vi "MGI Set Multicolumn Listbox Scrollbar.vi"(10 "Error In":errorcluster, 11 "Listbox Reference In":refnum<vi>) -> (2 "Error Out":errorcluster, 3 "Listbox Reference Out":refnum<vi>)   [LabVIEW 2016]
doc: "Show or hide the specified multicolumn listbox's horizontal and vertical scrollbar based on the listbox contents. This VI will also set the scrollbar position as necessary to ensure that some of the listbox's contents is displayed.\n\nAuthored by Shawn Walpole\nsupport@mooregoodideas.com\nwww.mooregoodideas.com\n\nCopyright (c) 2010, Moore Good Ideas, Inc.\n\nAll rights reserved.\n\nRedistribution and use in source and binary forms, with or without modification, are permitted provided that the following conditions are met:\n\n * Redistributions of source code must retain the above copyright notice, this list of conditions and the following disclaimer.\n * Redistributions in binary form must reproduce the above copyright notice, this list of conditions and the following disclaimer in the documentation and/or other materials provided with the distribution.\n * Neither the name of Moore Good Ideas, Inc. nor the names of its contributors may be used to endorse or promote products derived from this software without specific prior written permission.\n\nTHIS SOFTWARE IS PROVIDED BY THE COPYRIGHT HOLDERS AND CONTRIBUTORS \"AS IS\" AND ANY EXPRESS OR IMPLIED WARRANTIES, INCLUDING, BUT NOT LIMITED TO, THE IMPLIED WARRANTIES OF MERCHANTABILITY AND FITNESS FOR A PARTICULAR PURPOSE ARE DISCLAIMED. IN NO EVENT SHALL THE COPYRIGHT OWNER OR CONTRIBUTORS BE LIABLE FOR ANY DIRECT, INDIRECT, INCIDENTAL, SPECIAL, EXEMPLARY, OR CONSEQUENTIAL DAMAGES (INCLUDING, BUT NOT LIMITED TO, PROCUREMENT OF SUBSTITUTE GOODS OR SERVICES; LOSS OF USE, DATA, OR PROFITS; OR BUSINESS INTERRUPTION) HOWEVER CAUSED AND ON ANY THEORY OF LIABILITY, WHETHER IN CONTRACT, STRICT LIABILITY, OR TORT (INCLUDING NEGLIGENCE OR OTHERWISE) ARISING IN ANY WAY OUT OF THE USE OF THIS SOFTWARE, EVEN IF ADVISED OF THE POSSIBILITY OF SUCH DAMAGE."
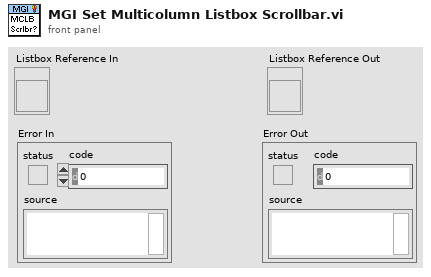
[diagram p1: front panel]
types:
  T1 = typedef "LVRowAndColumnUnsignedTypeDef.ctl" = cluster{"Row":u32, "Column":u32}
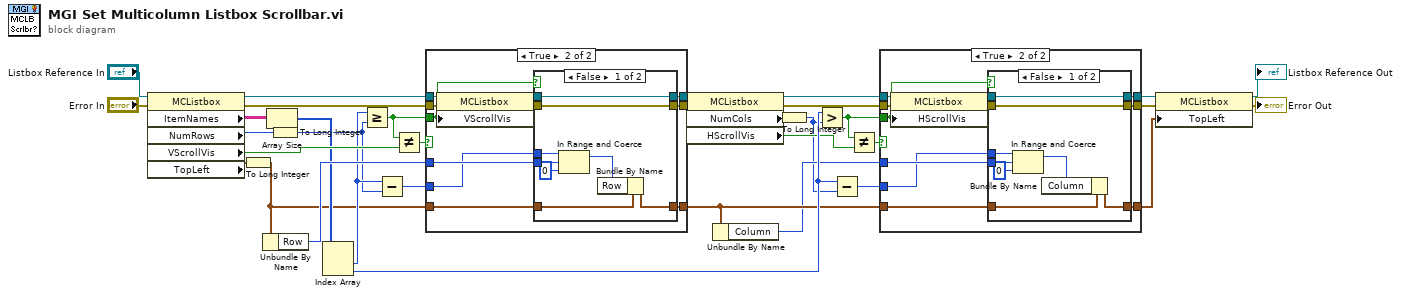
[diagram p0: block diagram]
diagram:
  n1 = property class="MCListbox"(reference="Listbox Reference In", error in="Error In") -> (reference out=w34:refnum<vi>, error out=w27:errorcluster, "ItemNames"=w32:string[][], "NumRows"=w4:u32, "VScrollVis"=w31:bool, "TopLeft"=w2:T1)
  n2 = To Long Integer(number=w2) -> (32bit integer=w1:cluster{"Row":i32, "Column":i32})
  n3 = Unbundle By Name(w1) -> ("Row"=w25:i32)
  n4 = Array Size(array=w32) -> (size(s)=w7:i32[])
  n5 = To Long Integer(number=w4) -> (32bit integer=w3:i32)
  n6 = Index Array(array=w7) -> (element #1=w24:i32, element #2=w22:i32)  [unwired: 2 in]
  n7 = Greater Or Equal?(x=w24, y=w3) -> (x >= y?=w30:bool)
  n8 = Subtract(x=w24, y=w3) -> (x-y=w26:i32)
  n9 = Not Equal?(x=w30, y=w31) -> (x != y?=w29:bool)
  n10 = case shown="True" w29 {
    tunnel: w34 -> [w37 w48]
    tunnel: w30 -> [_ w42]
    tunnel: [w37 w44] -> w18
    tunnel: w27 -> [w36 w47]
    tunnel: [w36 w43] -> w16
    tunnel: w25 -> [_ w41]
    tunnel: w26 -> [_ w40]
    tunnel: w1 -> [w35 w39]
    tunnel: [w35 w38] -> w20
    frame False {
    }
    frame True {
      n11 = property class="MCListbox"(reference=w48, error in=w47, "VScrollVis"=w42) -> (reference out=w46:refnum<vi>, error out=w45:errorcluster)
      n12 = case shown="False" w42 {
        tunnel: w46 -> [w51 w59]
        tunnel: w45 -> [w52 w58]
        tunnel: [w51 w59] -> w44
        tunnel: [w52 w58] -> w43
        tunnel: w41 -> [w56 _]
        tunnel: w40 -> [w54 _]
        tunnel: w39 -> [w53 w57]
        tunnel: [w49 w57] -> w38
        frame False {
          n13 = In Range and Coerce(upper limit=w54, x=w56, lower limit=0) -> (coerced(x)=w50:i32)  [unwired: 1 out]
          n14 = Bundle By Name(cluster=w53, "Row"=w50) -> (w49:cluster{"Row":i32, "Column":i32})
        }
        frame True {
        }
      }
    }
  }
  n15 = property class="MCListbox"(reference=w18, error in=w16) -> (reference out=w19:refnum<vi>, error out=w17:errorcluster, "NumCols"=w6:u32, "HScrollVis"=w14:bool)
  n16 = Unbundle By Name(w20) -> ("Column"=w15:i32)
  n17 = To Long Integer(number=w6) -> (32bit integer=w5:i32)
  n18 = Greater?(x=w22, y=w5) -> (0:w13:bool)
  n19 = Subtract(x=w22, y=w5) -> (x-y=w21:i32)
  n20 = Not Equal?(x=w13, y=w14) -> (x != y?=w23:bool)
  n21 = case shown="True" w23 {
    tunnel: w19 -> [w62 w73]
    tunnel: w13 -> [_ w67]
    tunnel: [w62 w69] -> w9
    tunnel: w17 -> [w61 w72]
    tunnel: [w61 w68] -> w10
    tunnel: w15 -> [_ w66]
    tunnel: w21 -> [_ w65]
    tunnel: w20 -> [w60 w64]
    tunnel: [w60 w63] -> w8
    frame False {
    }
    frame True {
      n22 = property class="MCListbox"(reference=w73, error in=w72, "HScrollVis"=w67) -> (reference out=w71:refnum<vi>, error out=w70:errorcluster)
      n23 = case shown="False" w67 {
        tunnel: w71 -> [w76 w84]
        tunnel: w70 -> [w77 w83]
        tunnel: [w76 w84] -> w69
        tunnel: [w77 w83] -> w68
        tunnel: w66 -> [w81 _]
        tunnel: w65 -> [w79 _]
        tunnel: w64 -> [w78 w82]
        tunnel: [w74 w82] -> w63
        frame False {
          n24 = In Range and Coerce(upper limit=w79, x=w81, lower limit=0) -> (coerced(x)=w75:i32)  [unwired: 1 out]
          n25 = Bundle By Name(cluster=w78, "Column"=w75) -> (w74:cluster{"Row":i32, "Column":i32})
        }
        frame True {
        }
      }
    }
  }
  n26 = property class="MCListbox"(reference=w9, error in=w10, "TopLeft"=w8) -> (reference out=→"Listbox Reference Out":refnum<vi>, error out=→"Error Out":errorcluster)
